vi "MPU6050.vi"() -> ()   [LabVIEW 2014]
uses:
  <vilib>/MakerHub/LINX/Public/Sensors/Accelerometer/MPU60X0/DeviceAddresses.ctl
  <vilib>/MakerHub/LINX/Public/Sensors/Accelerometer/MPU60X0/Clock Source.ctl
  <vilib>/MakerHub/LINX/Public/Sensors/Accelerometer/MPU60X0/GyroFullScaleRanges.ctl
  <vilib>/MakerHub/LINX/Public/Sensors/Accelerometer/MPU60X0/AccelFullScaleRanges.ctl
  <vilib>/MakerHub/LINX/Public/Utilities/Open Serial.vi
  <vilib>/MakerHub/LINX/LMH-LINX.lvlib
  <vilib>/MakerHub/LINX/Public/Sensors/Accelerometer/MPU60X0/MPU60X0.lvlib
panel:
  in  "CONNECT":bool
  out "Gyro  Data (dps)":T1
  out "Acceleration Data (g)":T1
  out "Thermometer":dbl(slide) scale=0.0..100.0
  out "Temperature (°C)":dbl
  in  "Accel Full Scale Range":T2
  in  "Gyro Full Scale Range":T3
  in  "I2C Channel":u8
  in  "Clock Source":T4
  in  "I2C Slave Address":T5=enum."0x69"
  in  "STOP":bool
  in  "Serial Port":refnum<visa-resource-name>="N/A"
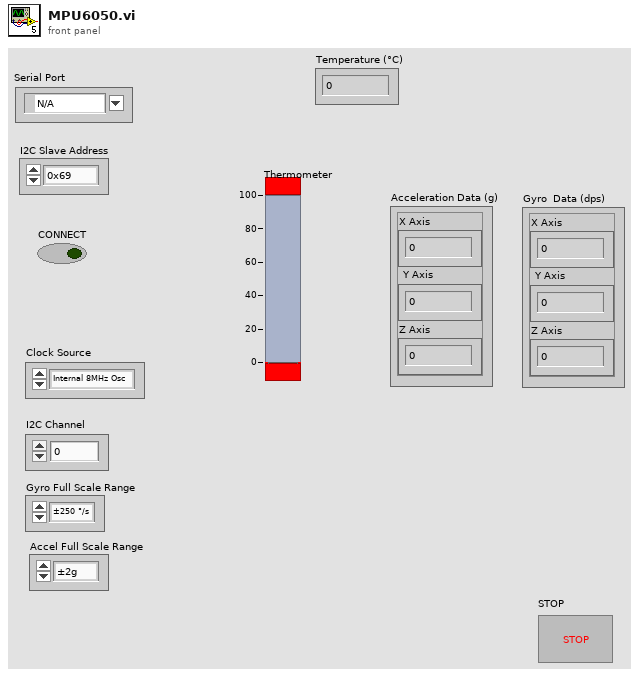
[diagram p1: front panel]
types:
  T1 = cluster{"X Axis":i16, "Y Axis":i16, "Z Axis":i16}
  T2 = typedef "LMH-LINX.lvlib/MPU60X0.lvlib/AccelFullScaleRanges.ctl" = enum16{"±2g", "±4g", "±8g", "±16g"}
  T3 = typedef "LMH-LINX.lvlib/MPU60X0.lvlib/GyroFullScaleRanges.ctl" = enum8{"±250 °/s", "±500 °/s", "±1000 °/s", "±2000 °/s"}
  T4 = typedef "LMH-LINX.lvlib/MPU60X0.lvlib/Clock Source.ctl" = enum8{"Internal 8MHz Osc", "PLL with X Gyro Ref", "PLL with Y Gyro Ref", "PLL with Z Gyro Ref", "PLL with ext 32.768 KHz Ref", "PLL with ext 19.2 MHz Ref", "Reserved", "Hold in reset"}
  T5 = typedef "LMH-LINX.lvlib/MPU60X0.lvlib/DeviceAddresses.ctl" = enum16{"0x68", "0x69"}
  T6 = typedef "LMH-LINX.lvlib/LINX Ref.ctl" = cluster{"IO":T7, "Interface":T8, "LINX Device Config":T9}
  T7 = typedef "LMH-LINX.lvlib/Platform.ctl" = enum16{"Remote", "Local"}
  T8 = typedef "LMH-LINX.lvlib/Interface.ctl" = enum16{"Serial", "TCP"}
  T9 = typedef "LMH-LINX.lvlib/Device.lvlib/LINX Device Config.ctl" = cluster{"Interface":T8, "COM Port":refnum<visa-resource-name>, "TCP Configuration":T10, "Device Family":u8, "Device ID":u8, "Device Name":string, "TCP Ref":refnum<k5>, "Channels":T11}
  T10 = typedef "LMH-LINX.lvlib/Device.lvlib/TCP Config.ctl" = cluster{"IP Address":string, "Port":u16}
  T11 = typedef "LMH-LINX.lvlib/Channels.ctl" = cluster{"DI":u8[], "DO":u8[], "AI":u8[], "AO":u8[], "PWM":u8[], "QE":u8[], "UART":u8[], "I2C 2":u8[], "SPI":u8[], "CAN":u8[], "Servo":u8[], "AI Ref (V)":dbl, "AI Resolution (Bits)":u8, "AO Ref (V)":dbl, "AO Resolution (Bits)":u8}
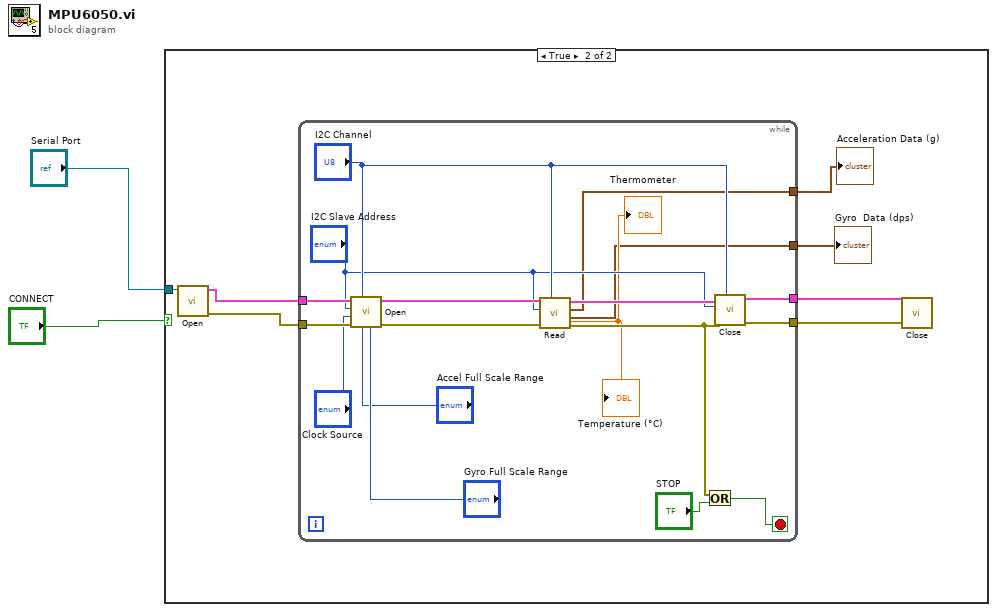
[diagram p0: block diagram]
diagram:
  n1 = case shown="True" "CONNECT" {
    tunnel: "Serial Port" -> [_ w9]
    frame False {
    }
    frame True {
      n2 = call-poly <vilib>:"Open.vi"("Serial Port"=w9) -> ("Error Out"=w6:errorcluster, "LINX Resource"=w8:T6)  [unwired: 8 in, 1 out]
      n3 = while {
        tunnel: w8 -> [w26]
        tunnel: [w23] -> w7
        tunnel: w6 -> [w22]
        tunnel: [w20] -> w5
        tunnel: [w11] -> w4
        tunnel: [w10] -> w3
        stop <- w27 stop-if-true
        n4 = call <vilib>:"Open.vi"("Gyro Full Scale Range"="Gyro Full Scale Range", "Accel Full Scale Range"="Accel Full Scale Range", "I2C Channel"="I2C Channel", "Error In"=w22, "Clock Source"="Clock Source", "I2C Slave Address"="I2C Slave Address", "LINX Resource"=w26) -> ("Error Out"=w21:errorcluster, "LINX Resource"=w25:T6)  [unwired: 3 in]
        n5 = call <vilib>:"Read.vi"("I2C Channel"="I2C Channel", "Error In"=w21, "I2C Slave Address"="I2C Slave Address", "LINX Resource"=w25) -> ("Error Out"=w19:errorcluster, "Gyro  Data (dps)"=w10:T1, "Acceleration Data (g)"=w11:T1, "LINX Resource"=w24:T6, "Temperature (°C)"=→"Temperature (°C)" →"Thermometer":dbl)  [unwired: 3 in]
        n6 = Or(x=w19, y="STOP") -> (x .or. y?=w27:bool)
        n7 = call <vilib>:"Close.vi"("I2C Channel (0)"="I2C Channel", "Error In"=w19, "I2C Slave Address (0)"="I2C Slave Address", "LINX Resource"=w24) -> ("Error Out"=w20:errorcluster, "LINX Resource"=w23:T6)  [unwired: 6 in]
      }
      "Acceleration Data (g)" <- w4
      "Gyro  Data (dps)" <- w3
      n8 = call <vilib>:"Close.vi"("Error In"=w5, "LINX Resource"=w7) -> ()  [unwired: 9 in, 1 out]
    }
  }
